vi "Accept-Encodings.vi"(8 "error in (no error)":errorcluster, 11 "Request in":refnum<class "Request.lvclass">) -> (0 "error out":errorcluster, 2 "Accept-Encodings":string[](array[string]), 3 "Request out":refnum<class "Request.lvclass">)   [LabVIEW 2020, in "HTTP Utils.lvlib" / "Request.lvclass"]
uses:
  Request.lvclass
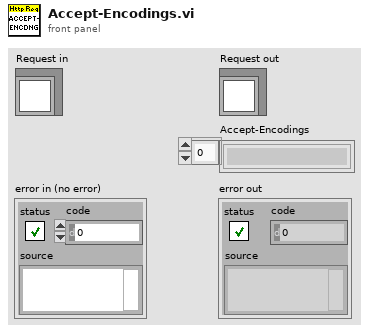
[diagram p1: front panel]
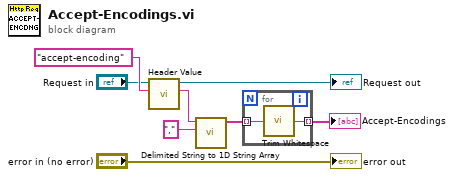
[diagram p0: block diagram]
diagram:
  n1 = call "Header Value.vi"("Header"="accept-encoding", "Request in"="Request in") -> ("Value"=w6:string, "Request out"=→"Request out":refnum<class "Request.lvclass">)  [unwired: 6 in, 2 out]
  n2 = call <vilib>:"Delimited String to 1D String Array.vi"("delimiter"=",", "delimited string"=w6) -> ("string array"=w2:string[])  [unwired: 9 in]
  n3 = for {
    tunnel: w2 -> [w10] mode=indexing
    tunnel: [w9] -> w1 mode=indexing
    n4 = call <vilib>:"Trim Whitespace.vi"("string"=w10) -> ("trimmed string"=w9:string)  [unwired: 1 in]
  }
  "Accept-Encodings" <- w1
  "error out" <- "error in (no error)"
